vi "Check string represents a number.vi"(7 "String":string) -> (6 "Is a number":bool, 8 "Number":dbl)   [LabVIEW 2019]
uses:
  <vilib>/regexp/Match Regular Expression.xnode
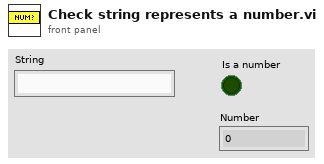
[diagram p1: front panel]
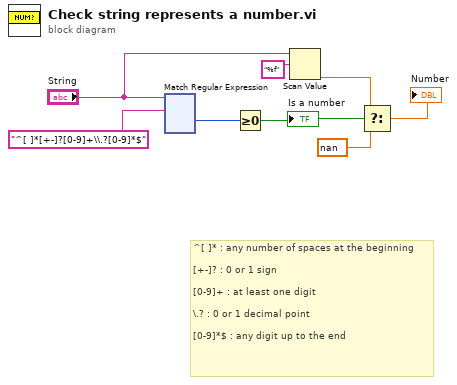
[diagram p0: block diagram]
diagram:
  # "^[ ]* : any number of spaces at the beginning\n\n[+-]? : 0 or 1 sign\n\n[0-9]+ : at least one digit\n\n\\.? : 0 or 1 decimal point\n\n[0-9]*$ : any digit up to the end"
  n1 = xnode "Match Regular Expression"("input string"="String", "regular expression"="^[ ]*[+-]?[0-9]+\\.?[0-9]*$") -> ("offset past match"=w7:i32)  [unwired: 4 in, 4 out]
  n2 = Greater Or Equal To 0?(x=w7) -> (x >= 0?=w5:bool)
  "Is a number" <- w5
  n3 = Scan Value(string="String", format string="%f") -> (value=w2:dbl)  [unwired: 1 in, 1 out]
  n4 = Select(t=w2, s=w5, f=nan) -> (s? t:f=→"Number":dbl)
